vi "Replace all instances of given substring.vi"(2 "Substring 2 (replace with this)":string, 3 "Substring 1 (find and replace this)":string, 4 "String In":string) -> (0 "number of replacements":i32, 1 "String Out (all instances of substring 1 replaced with substring 2)":string)   [LabVIEW 2016, in "Error Manager.lvlib"]
doc: "Replaces all instances of a substring with another.\n\n<B>Example 1</B>\n<B>Inputs</B>\n String In = \"Hello World, Hello World, Hello World\"\n Substring 1 = \"World\"\n Substring 2 = \"Planet\"\n<B>Outputs</B>\n String Out = \"Hello Planet, Hello Planet, Hello Planet\"\n\n<B>Example 2</B>\n<B>Inputs</B>\n String In = \"John has scored 91%. John has achieved an A*\"\n Substring 1 = \"John\"\n Substring 2 = \"Mary\"\n<B>Outputs</B>\n String Out = \"Mary has scored 91%. Mary has achieved an A*\"\n\nPerformance: This VI is inlined to increase performance"
uses:
  Error Manager.lvlib
panel:
  # "Input\nInputs to the VI"
  # "Development\ncontrols/indicators useful for development and testing, but which are not outputs of the VI"
  # "Output\nOutputs of the VI"
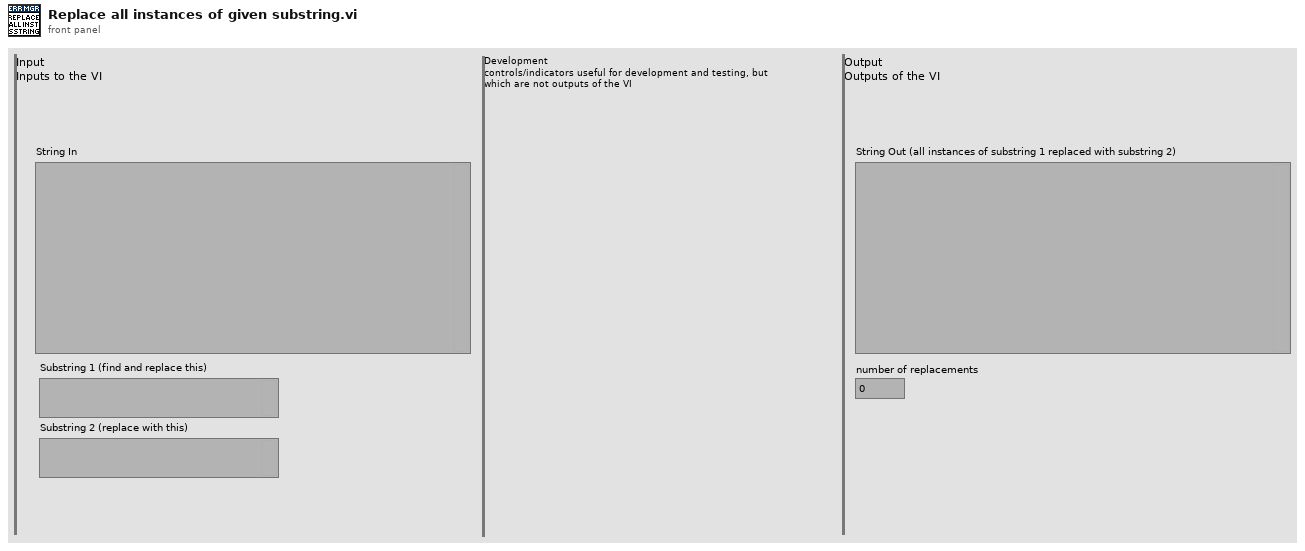
[diagram p1: front panel]
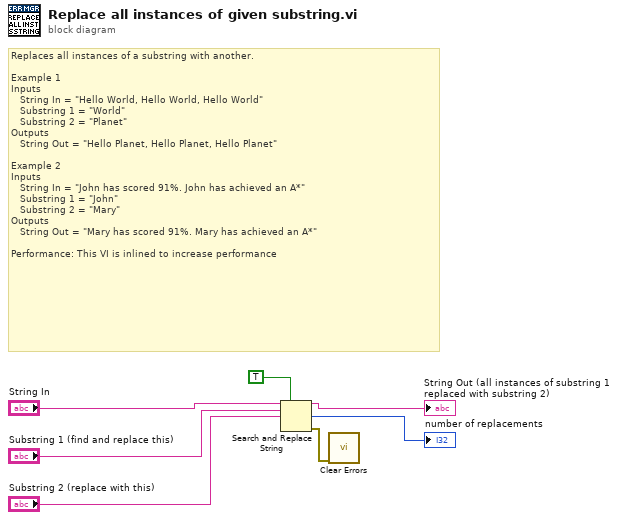
[diagram p0: block diagram]
diagram:
  # "Replaces all instances of a substring with another.\n\nExample 1\nInputs\n   String In = \"Hello World, Hello World, Hello World\"\n   Substring 1 = \"World\"\n   Substring 2 = \"Planet\"\nOutputs\n   String Out = \"Hello Planet, Hello Planet, Hello Planet\"\n\nExample 2\nInputs\n   String In = \"John has scored 91%. John has achieved an A*\"\n   Substring 1 = \"John\"\n   Substring 2 = \"Mary\"\nOutputs\n   String Out = \"Mary has scored 91%. Mary has achieved an A*\"\n\nPerformance: This VI is inlined to increase performance"
  n1 = Search and Replace String(replace all?=TRUE ("replace all? (F)"), input string="String In", search string="Substring 1 (find and replace this)", replace string="Substring 2 (replace with this)") -> (result string=→"String Out (all instances of substring 1 replaced with substring 2)":string, number of replacements=→"number of replacements":i32, error out=w1:errorcluster)  [unwired: 4 in, 1 out]
  n2 = call <vilib>:"Clear Errors.vi"("error in (no error)"=w1) -> ()  [unwired: 5 in, 2 out]
